vi "Proceed Menu Selection.vi"(8 "error in (no error)":errorcluster, 10 "MenuTag":string, 11 "HIJ Vision Camera App In":refnum<class "HIJ Vision Camera App.lvclass">) -> (0 "error out":errorcluster, 3 "HIJ Vision Camera App Out":refnum<class "HIJ Vision Camera App.lvclass">)   [LabVIEW 2020, in "HIJ Vision Camera App.lvlib" / "HIJ Vision Camera App.lvclass"]
uses:
  HIJ Vision Camera App.lvclass
  HIJ Vision Camera App.lvclass/HIJ Vision Camera App.ctl
  HIJ Vision Camera App Dialog/HIJ Vision Camera App Dialog/HIJ Vision Camera App Dialog.lvclass/HIJ Vision Camera App Dialog.ctl
  HIJ Vision Camera App Dialog/HIJ Vision Camera App Dialog/Read Camera Name.vi
  HIJ Vision Camera App Dialog/HIJ Vision Camera App Dialog/HIJ Vision Camera App Dialog.lvclass
  HIJ Vision Application/HIJ Vision Application/HIJ Vision Application.lvclass
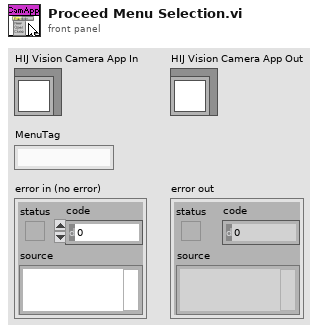
[diagram p1: front panel]
types:
  T1 = typedef "IMAQdx.ctl" = refnum<k21>
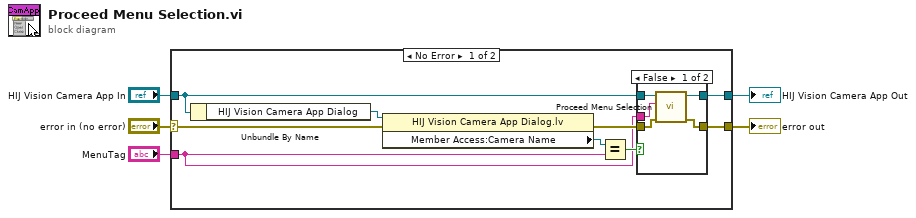
[diagram p0: block diagram]
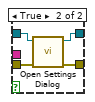
[diagram p2: hidden frame]
diagram:
  n1 = case shown="No Error" "error in (no error)" {
    selector: "error in (no error)" -> [w9 w25]
    tunnel: [w13 w25] -> w4
    tunnel: [w14 w24] -> w2
    tunnel: "HIJ Vision Camera App In" -> [w12 w24]
    tunnel: "MenuTag" -> [w6 _]
    frame No Error {
      n2 = Unbundle By Name(w12) -> ("HIJ Vision Camera App Dialog"=w11:refnum<class "HIJ Vision Camera App Dialog.lvclass">)
      n3 = property class="HIJ Vision Camera App Dialog.lv"(reference=w11, error in=w9) -> (error out=w8:errorcluster, "Member Access:Camera Name"=w10:T1)  [unwired: 1 out]
      n4 = Equal?(x=w10, y=w6) -> (x = y?=w7:bool)
      n5 = case shown="False" w7 {
        tunnel: [w18 w23] -> w14
        tunnel: [w16 w22] -> w13
        tunnel: w12 -> [w19 w21]
        tunnel: w8 -> [w17 w20]
        tunnel: w6 -> [w15 _]
        frame False {
          n6 = call-parent "Proceed Menu Selection.vi"("error in (no error)"=w17, "Menu Tag"=w15, "ViewableActor in"=w19) -> ("error out"=w16:errorcluster, "ViewableActor out"=w18:refnum<class "HIJ Vision Camera App.lvclass">)  [unwired: 7 in]
        }
        frame True {
          n7 = call "Open Settings Dialog.vi"("error in (no error)"=w20, "HIJ Vision Camera App in"=w21) -> ("error out"=w22:errorcluster, "HIJ Vision Camera App out"=w23:refnum<class "HIJ Vision Camera App.lvclass">)  [unwired: 8 in]
        }
      }
    }
    frame Error {
    }
  }
  "error out" <- w4
  "HIJ Vision Camera App Out" <- w2
